vi "SPI Engine Timer.vi"(11 "data rate (S/s)":u32=10000) -> (3 "Acq Loop Ticks":u32)   [LabVIEW 2014]
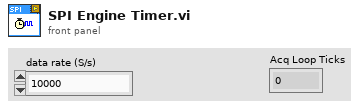
[diagram p1: front panel]
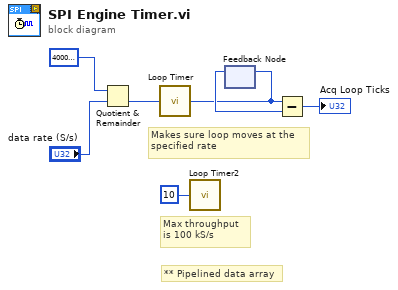
[diagram p0: block diagram]
diagram:
  # "Max throughput\nis 100 kS/s"
  # "Makes sure loop moves at the\nspecified rate"
  # "** Pipelined data array"
  n1 = Quotient & Remainder(x=u32 40000000 ("oclk freq"), y="data rate (S/s)") -> (floor(x/y)=w2:u32)  [unwired: 1 out]
  n2 = call "Loop Timer"("Count(Ticks)"=w2) -> ("Tick Count(Ticks)"=w6:u32)
  n3 = call "Loop Timer2"("Count(uSec)"=u8 10 ("Count(Ticks)")) -> ()  [unwired: 1 out]
  n4 = feedback #1() -> (w7:u32)  [unwired: 1 out]
  n5 = feedback-in #1(w6) -> ()
  n6 = Subtract(x=w6, y=w7) -> (x-y=→"Acq Loop Ticks":u32)
